vi "Init.vi"(8 "error in (no error)":errorcluster, 10 "isAddrLow(76)":bool, 11 "LINX Resource":T1) -> (0 "error out":errorcluster, 3 "BME680 out":refnum<class "BME680.lvclass">)   [LabVIEW 2022 SP3, in "BME680.lvlib" / "BME680.lvclass"]
uses:
  BME680.lvclass
  BME680.lvclass/BME680.ctl
  <vilib>/MakerHub/LINX/LMH-LINX.lvlib
  <vilib>/MakerHub/LINX/Private/Type Defs/Platform.ctl
  <vilib>/MakerHub/LINX/Private/Type Defs/Interface.ctl
  <vilib>/MakerHub/LINX/Private/Device/Type Defs/TCP Config.ctl
  <vilib>/MakerHub/LINX/Private/Device/Device.lvlib
  <vilib>/MakerHub/LINX/Private/Device/Type Defs/Channels.ctl
  <vilib>/MakerHub/LINX/Private/Device/Type Defs/LINX Device Config.ctl
  <vilib>/MakerHub/LINX/Private/Type Defs/LINX Ref.ctl
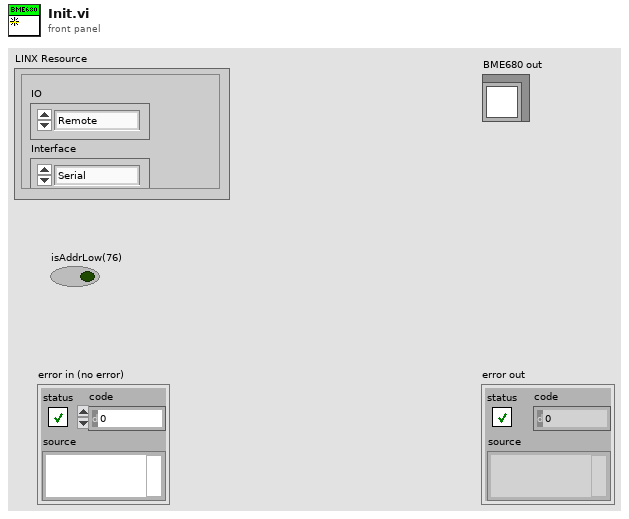
[diagram p1: front panel]
types:
  T1 = typedef "LMH-LINX.lvlib/LINX Ref.ctl" = cluster{"IO":T2, "Interface":T3, "LINX Device Config":T4}
  T2 = typedef "LMH-LINX.lvlib/Platform.ctl" = enum16{"Remote", "Local"}
  T3 = typedef "LMH-LINX.lvlib/Interface.ctl" = enum16{"Serial", "TCP"}
  T4 = typedef "LMH-LINX.lvlib/Device.lvlib/LINX Device Config.ctl" = cluster{"Interface":T3, "COM Port":refnum<visa-resource-name>, "TCP Configuration":T5, "Device Family":u8, "Device ID":u8, "Device Name":string, "TCP Ref":refnum<k5>, "Channels":T6}
  T5 = typedef "LMH-LINX.lvlib/Device.lvlib/TCP Config.ctl" = cluster{"IP Address":string, "Port":u16}
  T6 = typedef "LMH-LINX.lvlib/Channels.ctl" = cluster{"DI":u8[], "DO":u8[], "AI":u8[], "AO":u8[], "PWM":u8[], "QE":u8[], "UART":u8[], "I2C 2":u8[], "SPI":u8[], "CAN":u8[], "Servo":u8[], "AI Ref (V)":dbl, "AI Resolution (Bits)":u8, "AO Ref (V)":dbl, "AO Resolution (Bits)":u8}
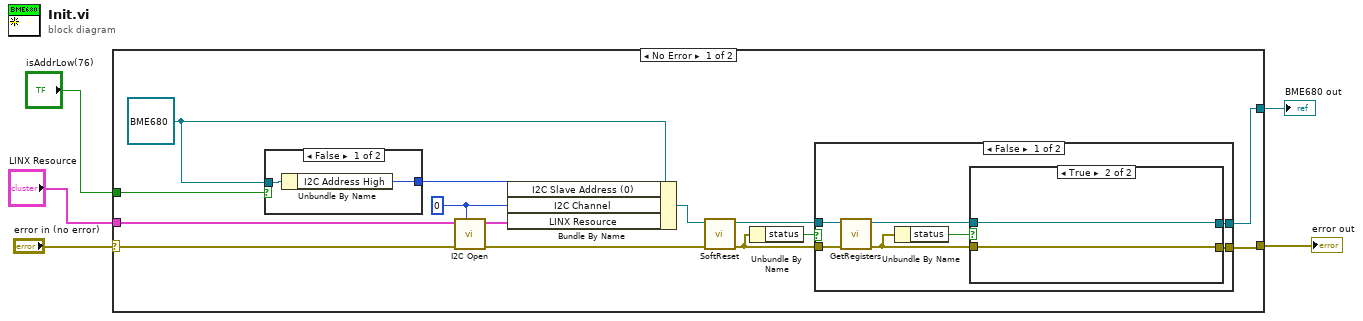
[diagram p0: block diagram]
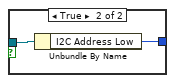
[diagram p2: hidden frame]
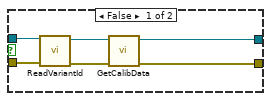
[diagram p3: hidden frame]
diagram:
  n1 = case shown="No Error" "error in (no error)" {
    selector: "error in (no error)" -> [w10 w41]
    tunnel: [w11 w41] -> w4
    tunnel: [w18 _] -> w3
    tunnel: "isAddrLow(76)" -> [w17 _]
    tunnel: "LINX Resource" -> [w8 _]
    frame No Error {
      w6 = u8 0 ("Linx I2C.I2C Channel")
      w16 = refnum<class "BME680.lvclass"> refnum ("BME680 in")
      n2 = case shown="False" w17 {
        tunnel: w16 -> [w21 w23]
        tunnel: [w20 w22] -> w15
        frame False {
          n3 = Unbundle By Name(w21) -> ("I2C Address High"=w20:u8)
        }
        frame True {
          n4 = Unbundle By Name(w23) -> ("I2C Address Low"=w22:u8)
        }
      }
      n5 = call <vilib>:"I2C Open.vi"("I2C Channel (0)"=w6, "Error In"=w10, "LINX Resource"=w8) -> ("Error Out"=w9:errorcluster, "LINX Resource"=w7:T1)  [unwired: 7 in]
      n6 = Bundle By Name(cluster=w16, "I2C Slave Address (0)"=w15, "I2C Channel"=w6, "LINX Resource"=w7) -> (w14:refnum<class "BME680.lvclass">)
      n7 = call-dynamic "SoftReset.vi"("error in (no error)"=w9, "BME680 in"=w14) -> ("error out"=w13:errorcluster, "BME680 out"=w19:refnum<class "BME680.lvclass">)  [unwired: 8 in]
      n8 = Unbundle By Name(w13) -> ("status"=w12:bool)
      n9 = case shown="False" w12 {
        tunnel: w19 -> [w30 w39]
        tunnel: w13 -> [w29 w40]
        tunnel: [w28 w39] -> w18
        tunnel: [w24 w40] -> w11
        frame False {
          n10 = call-dynamic "GetRegisters.vi"("error in (no error)"=w29, "BME680 in"=w30) -> ("error out"=w27:errorcluster, "BME680 out"=w26:refnum<class "BME680.lvclass">)  [unwired: 7 in, 1 out]
          n11 = Unbundle By Name(w27) -> ("status"=w25:bool)
          n12 = case shown="True" w25 {
            tunnel: w27 -> [w36 w37]
            tunnel: [w34 w38] -> w28
            tunnel: w26 -> [w33 w38]
            tunnel: [w31 w37] -> w24
            frame False {
              n13 = call "ReadVariantId.vi"("error in (no error)"=w36, "BME68x in"=w33) -> ("error out"=w35:errorcluster, "BME68x out"=w32:refnum<class "BME680.lvclass">)  [unwired: 8 in]
              n14 = call "GetCalibData.vi"("error in (no error)"=w35, "BME68x in"=w32) -> ("error out"=w31:errorcluster, "BME68x out"=w34:refnum<class "BME680.lvclass">)  [unwired: 8 in]
            }
            frame True {
            }
          }
        }
        frame True {
        }
      }
    }
    frame Error {
    }
  }
  "error out" <- w4
  "BME680 out" <- w3
